vi "createDeviceData.vi"(8 "error in (no error)":errorcluster, 11 "AoDeviceData in":refnum<class "AoDeviceData.lvclass">) -> (0 "error out":errorcluster, 3 "AoDeviceData out":refnum<class "AoDeviceData.lvclass">)   [LabVIEW 2009, in "DataMappers.lvlib" / "AoDeviceData.lvclass"]
uses:
  AoDeviceData.lvclass
  Hal/Channels/VoltOutput/AnalogOutput.lvclass
  AoDeviceData.lvclass/AoDeviceData.ctl
  DeviceData.lvclass
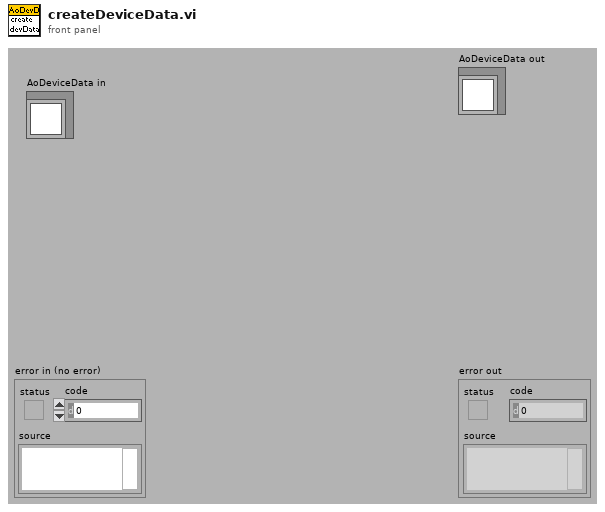
[diagram p1: front panel]
types:
  T1 = cluster{"Clock source":string, "Clock rate":dbl, "Start trigger line":string, "Sample Rate":dbl, "Sample No.":dbl}
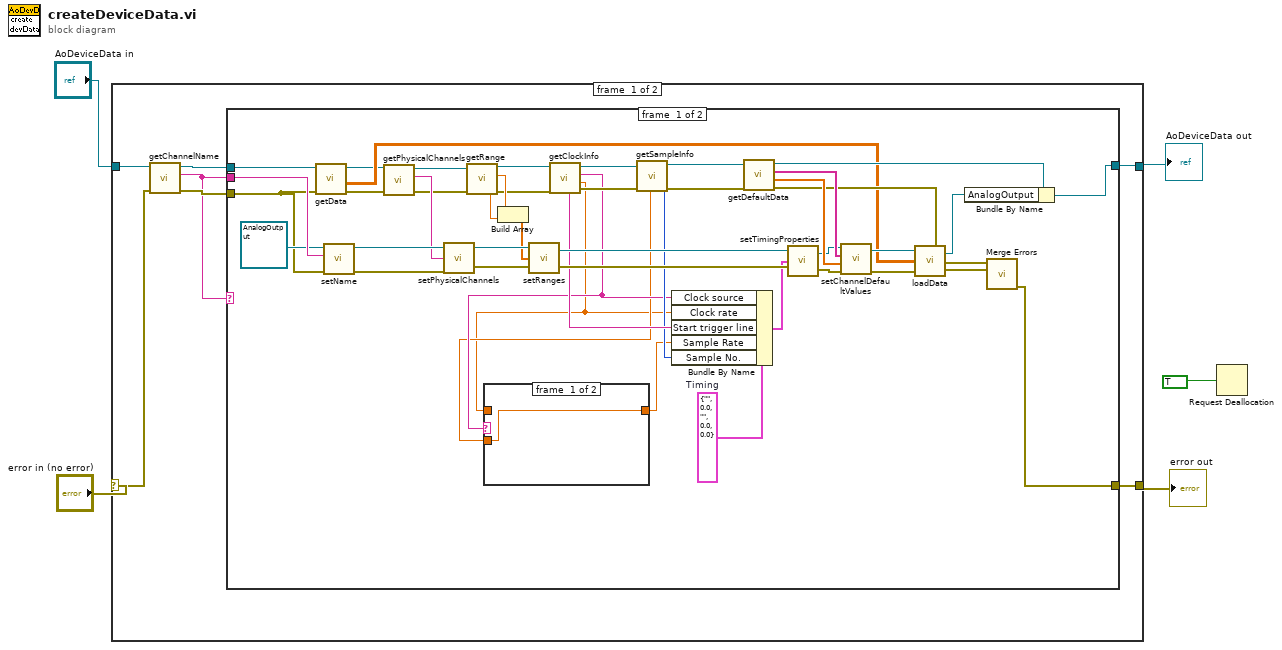
[diagram p0: block diagram]
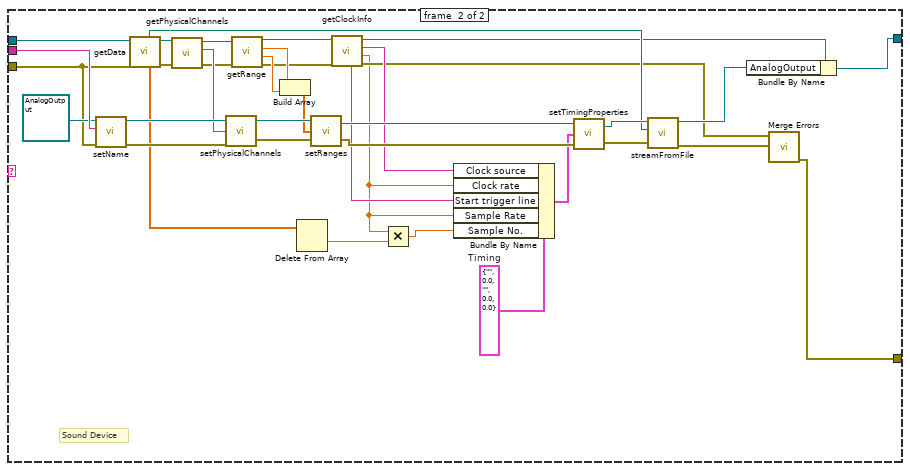
[diagram p3: hidden frame]
diagram:
  n1 = case shown="No Error" "error in (no error)" {
    selector: "error in (no error)" -> [w11 w97]
    tunnel: [w9 w98] -> w2
    tunnel: "AoDeviceData in" -> [w12 w98]
    tunnel: [w10 w97] -> w3
    frame #0 {
      n2 = call "getChannelName.vi"("error in (no error)"=w11, "DeviceData in"=w12) -> ("error out"=w7:errorcluster, "channelName"=w6:string, "DeviceData out"=w8:refnum<class "AoDeviceData.lvclass">)  [unwired: 7 in]
      n3 = case shown="Default" w6 {
        tunnel: w6 -> [w57 w96]
        tunnel: [w27 w76] -> w10
        tunnel: [w26 w66] -> w9
        tunnel: w8 -> [w21 w73]
        tunnel: w7 -> [w20 w74]
        frame #0 {
          w39 = T1 {"Clock source"="", "Clock rate"=0.0, "Start trigger line"="", "Sample Rate"=0.0, "Sample No."=0.0}  # Timing
          n4 = call "getData.vi"("error in (no error)"=w20, "DeviceData in"=w21) -> ("error out"=w22:errorcluster, "dataArray"=w19:dbl[][], "DeviceData out"=w18:refnum<class "AoDeviceData.lvclass">)  [unwired: 4 in, 3 out]
          n5 = call "setName.vi"("error in (no error)"=w20, "name"=w57, "AnalogOutput.lvclass in"=refnum<class "AnalogOutput.lvclass"> refnum ("Hardware:Channels.lvlib:AnalogOutput.lvclass")) -> ("error out"=w54:errorcluster, "AnalogOutput.lvclass out"=w55:refnum<class "AnalogOutput.lvclass">)  [unwired: 7 in]
          n6 = call "getPhysicalChannels.vi"("error in (no error)"=w22, "DeviceData in"=w18) -> ("error out"=w49:errorcluster, "physicalChannels"=w53:string, "DeviceData out"=w50:refnum<class "AoDeviceData.lvclass">)  [unwired: 7 in]
          n7 = call-dynamic "setPhysicalChannels.vi"("error in (no error)"=w54, "Physical Channels"=w53, "AnalogOutput.lvclass in"=w55) -> ("error out"=w51:errorcluster, "AnalogOutput.lvclass out"=w52:refnum<class "AnalogOutput.lvclass">)
          n8 = call "getRange.vi"("error in (no error)"=w49, "AoDeviceData in"=w50) -> ("error out"=w44:errorcluster, "max"=w48:dbl, "min"=w47:dbl, "AoDeviceData out"=w45:refnum<class "AoDeviceData.lvclass">)  [unwired: 6 in]
          n9 = Build Array(w47, w48) -> (w46:dbl[])
          n10 = call "setRanges.vi"("error in (no error)"=w51, "Ranges"=w46, "AnalogOutput.lvclass in"=w52) -> ("error out"=w42:errorcluster, "AnalogOutput.lvclass out"=w43:refnum<class "AnalogOutput.lvclass">)
          n11 = call "getClockInfo.vi"("error in (no error)"=w44, "DeviceData in"=w45) -> ("error out"=w40:errorcluster, "masterClockRate"=w14:dbl, "clock"=w16:string, "DeviceData out"=w41:refnum<class "AoDeviceData.lvclass">, "start_trigger"=w38:string)  [unwired: 5 in]
          n12 = call-dynamic "getSampleInfo.vi"("error in (no error)"=w40, "DeviceData in"=w41) -> ("error out"=w35:errorcluster, "sampleRate"=w15:dbl, "sampleNumber"=w17:i32, "DeviceData out"=w36:refnum<class "AoDeviceData.lvclass">)  [unwired: 6 in]
          n13 = case shown="\"internal\"" w16 {
            tunnel: w15 -> [w58 _]
            tunnel: w14 -> [_ w59]
            tunnel: [w58 w59] -> w13
            frame #0 {
            }
            frame #1 {
            }
          }
          n14 = Bundle By Name(cluster=w39, "Clock source"=w16, "Clock rate"=w14, "Start trigger line"=w38, "Sample Rate"=w13, "Sample No."=w17) -> (w37:T1)
          n15 = call "getDefaultData.vi"("error in (no error)"=w35, "DeviceData in"=w36) -> ("error out"=w23:errorcluster, "calibratedValues"=w32:dbl[], "channelAddresses"=w33:string[], "DeviceData out"=w24:refnum<class "AoDeviceData.lvclass">)  [unwired: 6 in]
          n16 = call "setTimingProperties.vi"("error in (no error)"=w42, "Timing"=w37, "AnalogOutput.lvclass in"=w43) -> ("error out"=w34:errorcluster, "AnalogOutput.lvclass out"=w31:refnum<class "AnalogOutput.lvclass">)
          n17 = call "setChannelDefaultValues.vi"("error in (no error)"=w34, "calibratedValues"=w32, "channel_addresses"=w33, "AnalogOutput in"=w31) -> ("error out"=w29:errorcluster, "AnalogOutput out"=w30:refnum<class "AnalogOutput.lvclass">)  [unwired: 6 in]
          n18 = call-dynamic "loadData.vi"("error in (no error)"=w29, "Data"=w19, "AnalogOutput in"=w30) -> ("error out"=w28:errorcluster, "AnalogOutput out"=w25:refnum<class "AnalogOutput.lvclass">)
          n19 = Bundle By Name(cluster=w24, "AnalogOutput"=w25) -> (w26:refnum<class "AoDeviceData.lvclass">)
          n20 = call <vilib>:"Merge Errors.vi"("error in 2 (no error)"=w28, "error in 1 (no error)"=w23) -> ("error out"=w27:errorcluster)  [unwired: 5 in]
        }
        frame #1 {
          w80 = T1 {"Clock source"="", "Clock rate"=0.0, "Start trigger line"="", "Sample Rate"=0.0, "Sample No."=0.0}  # Timing
          # "Sound Device"
          n21 = call "setName.vi"("error in (no error)"=w74, "name"=w96, "AnalogOutput.lvclass in"=refnum<class "AnalogOutput.lvclass"> refnum ("Hardware:Channels.lvlib:AnalogOutput.lvclass")) -> ("error out"=w93:errorcluster, "AnalogOutput.lvclass out"=w94:refnum<class "AnalogOutput.lvclass">)  [unwired: 7 in]
          n22 = call "getData.vi"("error in (no error)"=w74, "DeviceData in"=w73) -> ("error out"=w75:errorcluster, "DeviceData out"=w72:refnum<class "AoDeviceData.lvclass">, "times"=w63:dbl[], "soundStreamPath"=w69:path)  [unwired: 4 in, 2 out]
          n23 = call "getPhysicalChannels.vi"("error in (no error)"=w75, "DeviceData in"=w72) -> ("error out"=w88:errorcluster, "physicalChannels"=w92:string, "DeviceData out"=w89:refnum<class "AoDeviceData.lvclass">)  [unwired: 7 in]
          n24 = call-dynamic "setPhysicalChannels.vi"("error in (no error)"=w93, "Physical Channels"=w92, "AnalogOutput.lvclass in"=w94) -> ("error out"=w90:errorcluster, "AnalogOutput.lvclass out"=w91:refnum<class "AnalogOutput.lvclass">)
          n25 = call "getRange.vi"("error in (no error)"=w88, "AoDeviceData in"=w89) -> ("error out"=w83:errorcluster, "max"=w87:dbl, "min"=w86:dbl, "AoDeviceData out"=w84:refnum<class "AoDeviceData.lvclass">)  [unwired: 6 in]
          n26 = Build Array(w86, w87) -> (w85:dbl[])
          n27 = Delete From Array(array=w63) -> (deleted portion=w61:dbl)  [unwired: 2 in, 1 out]
          n28 = call "setRanges.vi"("error in (no error)"=w90, "Ranges"=w85, "AnalogOutput.lvclass in"=w91) -> ("error out"=w81:errorcluster, "AnalogOutput.lvclass out"=w82:refnum<class "AnalogOutput.lvclass">)
          n29 = call "getClockInfo.vi"("error in (no error)"=w83, "DeviceData in"=w84) -> ("error out"=w65:errorcluster, "masterClockRate"=w62:dbl, "clock"=w79:string, "DeviceData out"=w67:refnum<class "AoDeviceData.lvclass">, "start_trigger"=w78:string)  [unwired: 5 in]
          n30 = Multiply(x=w62, y=w61) -> (x*y=w60:dbl)
          n31 = Bundle By Name(cluster=w80, "Clock source"=w79, "Clock rate"=w62, "Start trigger line"=w78, "Sample Rate"=w62, "Sample No."=w60) -> (w77:T1)
          n32 = call "setTimingProperties.vi"("error in (no error)"=w81, "Timing"=w77, "AnalogOutput.lvclass in"=w82) -> ("error out"=w70:errorcluster, "AnalogOutput.lvclass out"=w71:refnum<class "AnalogOutput.lvclass">)
          n33 = call-dynamic "streamFromFile.vi"("error in (no error)"=w70, "Path"=w69, "AnalogOutput in"=w71) -> ("error out"=w64:errorcluster, "AnalogOutput out"=w68:refnum<class "AnalogOutput.lvclass">)  [unwired: 7 in]
          n34 = Bundle By Name(cluster=w67, "AnalogOutput"=w68) -> (w66:refnum<class "AoDeviceData.lvclass">)
          n35 = call <vilib>:"Merge Errors.vi"("error in 2 (no error)"=w64, "error in 1 (no error)"=w65) -> ("error out"=w76:errorcluster)  [unwired: 5 in]
        }
      }
    }
    frame #1 {
    }
  }
  "error out" <- w3
  "AoDeviceData out" <- w2
  n36 = Request Deallocation(TRUE) -> ()
